vi "PID Controller.vi"(0 "setpoint":dbl, 1 "process variable":dbl, 2 "PID Gains":cluster{"Kp":dbl, "Ki":dbl, "Kd":dbl}, 3 "Reinitialize Integral":bool, 4 "Constrain":cluster{"Max Control":dbl, "Min Control":dbl}={"Max Control"=1.0, "Min Control"=-1.0}) -> (5 "Control Signal":dbl)   [LabVIEW 2016]
panel:
  out "Error":dbl(graph)
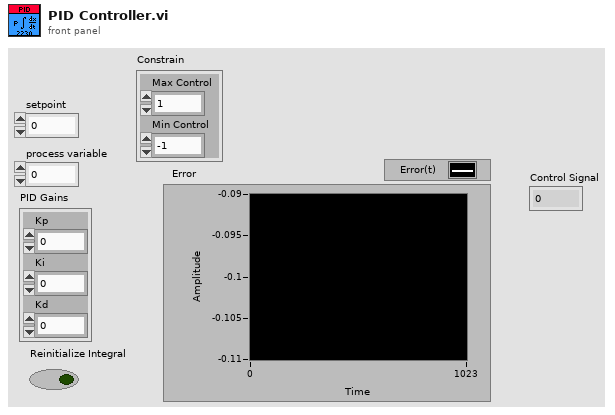
[diagram p1: front panel]
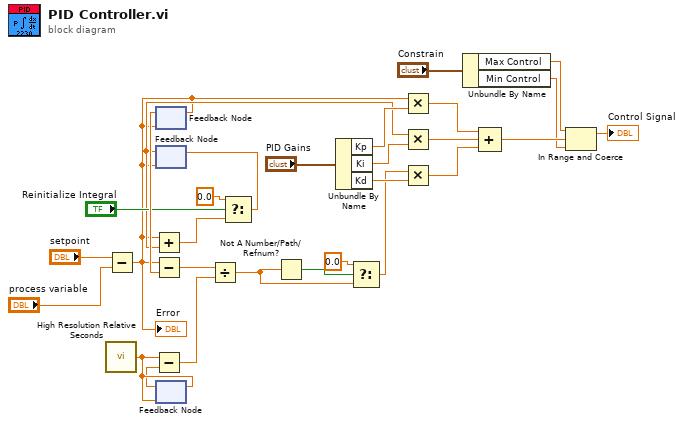
[diagram p0: block diagram]
diagram:
  n1 = call <vilib>:"High Resolution Relative Seconds.vi"() -> ("relative seconds"=w27:dbl)
  n2 = Subtract(x="setpoint", y="process variable") -> (x-y=w5:dbl)
  "Error" <- w5
  n3 = feedback #1(w5) -> (w23:dbl)
  n4 = Subtract(x=w5, y=w23) -> (x-y=w22:dbl)
  n5 = feedback-in #1(w5) -> ()
  n6 = feedback #2(w5) -> (w15:dbl)
  n7 = Add(x=w5, y=w15) -> (x+y=w16:dbl)
  n8 = feedback #3(w27) -> (w26:dbl)
  n9 = Subtract(x=w27, y=w26) -> (x-y=w21:dbl)
  n10 = feedback-in #3(w27) -> ()
  n11 = Divide(x=w22, y=w21) -> (x/y=w2:dbl)
  n12 = Select(t=0.0, s="Reinitialize Integral", f=w16) -> (s? t:f=w19:dbl)
  n13 = feedback-in #2(w19) -> ()
  n14 = Not A Number/Path/Refnum?(number/path/refnum=w2) -> (NaN/Path/Refnum?=w4:bool)
  n15 = Unbundle By Name("PID Gains") -> ("Kp"=w24:dbl, "Ki"=w14:dbl, "Kd"=w20:dbl)
  n16 = Select(t=0.0, s=w4, f=w2) -> (s? t:f=w1:dbl)
  n17 = Multiply(x=w5, y=w24) -> (x*y=w13:dbl)
  n18 = Multiply(x=w15, y=w14) -> (x*y=w12:dbl)
  n19 = Multiply(x=w1, y=w20) -> (x*y=w11:dbl)
  n20 = Unbundle By Name("Constrain") -> ("Max Control"=w8:dbl, "Min Control"=w7:dbl)
  n21 = Compound Arithmetic op=ADD(w13, w12, w11) -> (w10:dbl)
  n22 = In Range and Coerce(upper limit=w8, x=w10, lower limit=w7) -> (coerced(x)=→"Control Signal":dbl)  [unwired: 1 out]
